vi "Z-Scan-trigger.vi"(0 "trigger in":dbl[](array[numeric]), 1 "level":dbl=2.0, 3 "signal in":dbl[](array[numeric])=[0.0], 4 "trigger slope":u16(ring)=1 items=["Falling Edge", "Rising Edge"]) -> (5 "trigger out":dbl[](array[numeric]), 7 "signal out":dbl[](array[numeric]))   [LabVIEW 2014]
doc: "André Romero - 2016\nandretec@ifsc.usp.br"
uses:
  <vilib>/measure/mamon.llb/Trigger Detection for 1 Channel.vi
  <vilib>/measure/NI_MAPro.lvlib
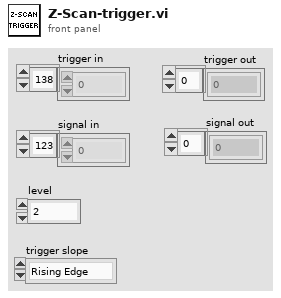
[diagram p1: front panel]
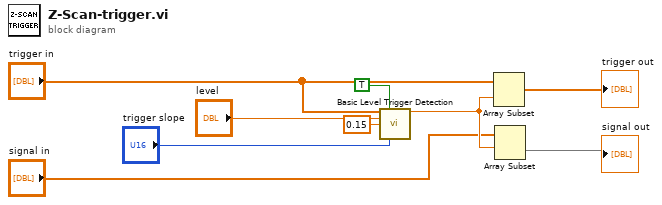
[diagram p0: block diagram]
diagram:
  n1 = call-poly <vilib>:"Basic Level Trigger Detection.vi"("signal in"="trigger in", "reset"=TRUE, "level"="level", "hysteresis"=0.15, "trigger slope"="trigger slope") -> ("trigger location"=w9:dbl)  [unwired: 8 in, 2 out]
  n2 = Array Subset(array="trigger in", index=w9) -> (→"trigger out":dbl[])  [unwired: 1 in]
  n3 = Array Subset(array="signal in", index=w9) -> (→"signal out":dbl[])  [unwired: 1 in]
